vi "Set Property.vi"(10 "Ctl Ref":refnum<vi>, 11 "Visible UIP In":refnum<class "VisibleUIP.lvclass">) -> (0 "Error Out":errorcluster, 3 "Visible UIP Out":refnum<class "VisibleUIP.lvclass">)   [LabVIEW 2020, in "UIM.lvlib" / "VisibleUIP.lvclass"]
uses:
  VisibleUIP.lvclass
  VisibleUIP.lvclass/VisibleUIP.ctl
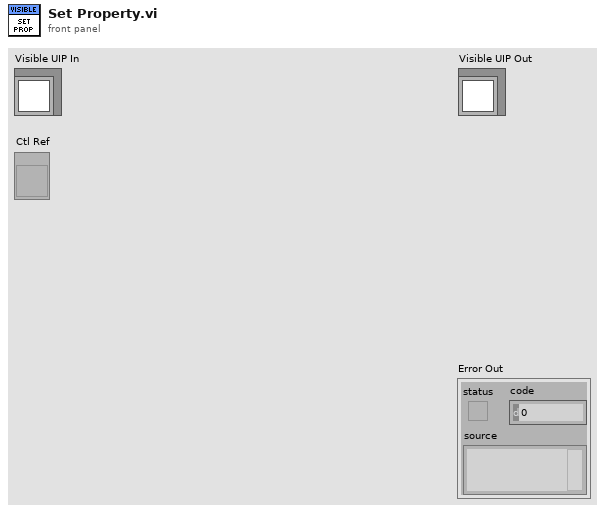
[diagram p1: front panel]
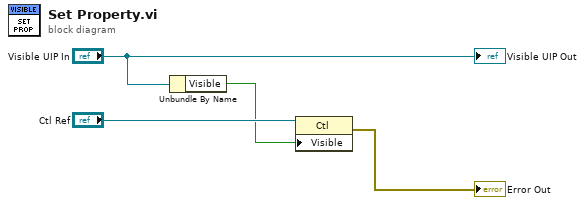
[diagram p0: block diagram]
diagram:
  n1 = Unbundle By Name("Visible UIP In") -> ("Visible"=w2:bool)
  n2 = property class="Ctl"(reference="Ctl Ref", "Visible"=w2) -> (error out=→"Error Out":errorcluster)  [unwired: 1 in, 1 out]
  "Visible UIP Out" <- "Visible UIP In"
